vi "Getlist_services.vi"(8 "error in (no error)":errorcluster, 11 "OneOfTemplate in":refnum<class "grpc_reflection_v1alpha_ServerReflectionRequest_message_request.lvclass">) -> (0 "error out":errorcluster, 2 "Get_Val":string, 3 "OneOfTemplate out":refnum<class "grpc_reflection_v1alpha_ServerReflectionRequest_message_request.lvclass">)   [LabVIEW 2019, in "reflection_server.lvlib" / "grpc_reflection_v1alpha_ServerReflectionRequest_message_request.lvclass"]
uses:
  grpc_reflection_v1alpha_ServerReflectionRequest_message_request.lvclass
  grpc_reflection_v1alpha_ServerReflectionRequest_message_request.lvclass/grpc_reflection_v1alpha_ServerReflectionRequest_message_request.ctl
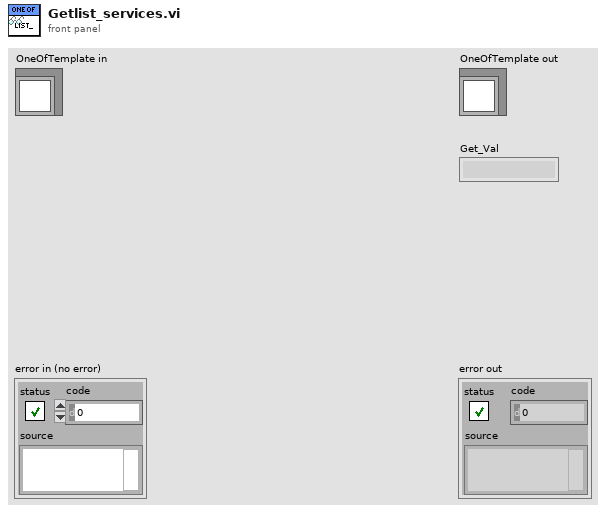
[diagram p1: front panel]
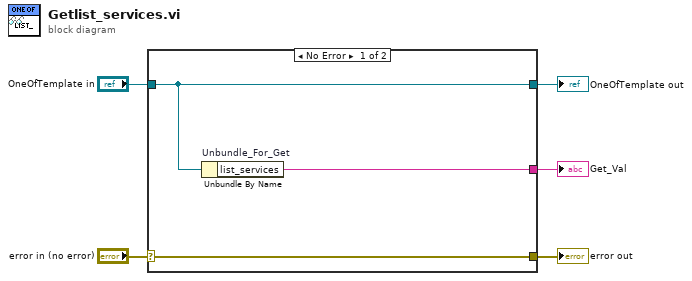
[diagram p0: block diagram]
diagram:
  n1 = case shown="No Error" "error in (no error)" {
    selector: "error in (no error)" -> [w8 w9]
    tunnel: [w8 w9] -> w4
    tunnel: [w7 w10] -> w2
    tunnel: "OneOfTemplate in" -> [w7 w10]
    tunnel: [w6 _] -> w1
    frame No Error {
      n2 = Unbundle By Name "Unbundle_For_Get"(w7) -> ("list_services"=w6:string)
    }
    frame Error {
    }
  }
  "error out" <- w4
  "OneOfTemplate out" <- w2
  "Get_Val" <- w1
